vi "communicateWithAnalyzer.vi"(8 "ErrorIn":errorcluster, 11 "QueuesIn":T1) -> (0 "ErrorOut":errorcluster, 3 "QueuesOut":T1)   [LabVIEW 2019]
uses:
  utilities/Queues.ctl
  GUIVIs/GUIOutput.ctl
  MobileAnalyzer/mainVIs/analyzeAccelerationDataVIs/AccelerationDataFrames.ctl
  MobileAnalyzer/mainVIs/analyzeAccelerationDataVIs/AnalyzedVibrationsData.ctl
  MobileAnalyzer/mainVIs/analyzeAccelerationDataVIs/calculateFaultIndicatorsVIs/FaultDetections.ctl
  MobileAnalyzer/mainVIs/analyzeAccelerationDataVIs/calculateFaultIndicatorsVIs/ParameterFaultDetection.ctl
  MobileAnalyzer/mainVIs/analyzeAccelerationDataVIs/calculateFaultIndicatorsVIs/FaultParameter.ctl
  MobileAnalyzer/mainVIs/analyzeAccelerationDataVIs/calculateFaultIndicatorsVIs/FrequencyFaultDetection.ctl
  masterVIs/Command.ctl
  MobileAnalyzer/mainVIs/TDMSmanagerVIs/TDMSAnalyzerData.ctl
  MobileAnalyzer/mainVIs/TDMSmanagerVIs/TDMSAnalyzerDataType.ctl
  communicateWithAnalyzerVIs/CommunicateWithAnalyzerState.ctl
  MobileAnalyzer/mainVIs/AmasterVIs/ACommand.ctl
  masterVIs/Thread.ctl
  <vilib>/dex/Stream Element Allocation Mode.ctl
  communicateWithAnalyzerVIs/ReceiverData.ctl
  communicateWithAnalyzerVIs/ReceiverDataType.ctl
  MobileAnalyzer/mainVIs/UIVIs/UIOutput.ctl
  communicateWithAnalyzerVIs/SenderData.ctl
  communicateWithAnalyzerVIs/SenderDataType.ctl
  MobileAnalyzer/mainVIs/utilities/FGVAction.ctl
panel:
  in  "Connect":bool
  in  "SenderConnected":bool
  in  "ReceiverConnected":bool
  in  "Exit":bool
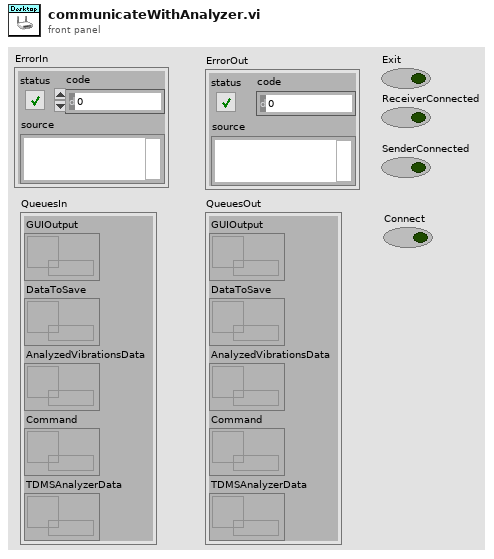
[diagram p1: front panel]
types:
  T1 = typedef "Queues.ctl" = cluster{"GUIOutput":refnum<queue>, "DataToSave":refnum<queue>, "AnalyzedVibrationsData":refnum<queue>, "Command":refnum<queue>, "TDMSAnalyzerData":refnum<queue>}
  T2 = typedef "ACommand.ctl" = enum16{"None", "Start", "Stop", "Restart", "SendFilesData", "DeleteAllData"}
  T3 = typedef "Command.ctl" = enum16{"None", "Connect", "Start", "Stop", "RestartAnalyzer", "Exit", "OpenDataFile", "CanBegin", "FileToSaveSettings", "AnalyzerSettings", "DownloadDataDialog", "DownloadData", "DeleteData"}
  T4 = typedef "Thread.ctl" = enum16{"GUI", "communicateWithAnalyzer", "saveDataToTDMS"}
  T5 = typedef "CommunicateWithAnalyzerState.ctl" = enum16{"Idle", "Connect", "Communicate", "Disconnect"}
  T6 = typedef "FGVAction.ctl" = enum16{"Read", "Write"}
  T7 = typedef "SenderDataType.ctl" = enum16{"Command", "AnalysisSettings"}
  T8 = typedef "SenderData.ctl" = cluster{"SenderDataType":T7, "Data":string}
  T9 = typedef "Stream Element Allocation Mode.ctl" = u32
  T10 = typedef "DesktopAppSettings.ctl" = cluster{"MobileAnalyzer IP":string, "Network Stream Timeout Code":i32, "Endpoint Destroyed Code":i32, "Save to file?":bool, "All threads":T4[], "Connected":bool, "AnalysisSettings":T11}
  T11 = typedef "AnalysisSettings.ctl" = cluster{"Fault Thresholds":T12, "Analysis series name":string, "Save data analysis?":bool}
  T12 = typedef "Thresholds.ctl" = cluster{"Parameters labels":T13[], "Parameters thresholds":dbl[], "Freqs and thresholds":dbl[][]}
  T13 = typedef "FaultParameter.ctl" = enum16{"Kurtosis", "RMS"}
  T14 = typedef "GUIOutput.ctl" = cluster{"Aquiring data":bool, "AnalyzerError":errorcluster, "FIFO overflow":bool, "Analyzing data":bool, "Connected":bool}
  T15 = typedef "ReceiverData.ctl" = cluster{"ReceiverDataType":T16, "Data":string}
  T16 = typedef "ReceiverDataType.ctl" = enum16{"UIOutput", "AnalyzedVibrationsData", "TDMSFiles"}
  T17 = typedef "UIOutput.ctl" = cluster{"Aquiring data":bool, "AnalyzerError":errorcluster, "FIFO overflow":bool, "Analyzing data":bool}
  T18 = typedef "AnalyzedVibrationsData.ctl" = cluster{"AccelerationDataFrames":T19, "Fault detections":T20}
  T19 = typedef "AccelerationDataFrames.ctl" = cluster{"AccelerationData":waveform(dbl)[], "Amplitudes":cluster{"f0":dbl, "df":dbl, "real part":dbl[]}[], "Phases":cluster{"f0":dbl, "df":dbl, "imaginary part":dbl[]}[]}
  T20 = typedef "FaultDetections.ctl" = cluster{"Parameters fault detection":T21[], "Frequencies fault detection":T22[]}
  T21 = typedef "ParameterFaultDetection.ctl" = cluster{"Axes Values":dbl[], "Axes Fault Detection":bool[], "Parameter Label":T13}
  T22 = typedef "FrequencyFaultDetection.ctl" = cluster{"Axes Values":dbl[], "Axes Fault Detection":bool[], "Frequency":dbl}
  T23 = typedef "TDMSAnalyzerData.ctl" = cluster{"TDMSAnalyzerDataType":T24, "group name out":string, "channel name(s) out":string[], "data":waveform(dbl)[], "File name":string}
  T24 = typedef "TDMSAnalyzerDataType.ctl" = enum16{"FileDataStart", "FileGroup", "FileDataStop", "NewFile", "EndOfFile"}
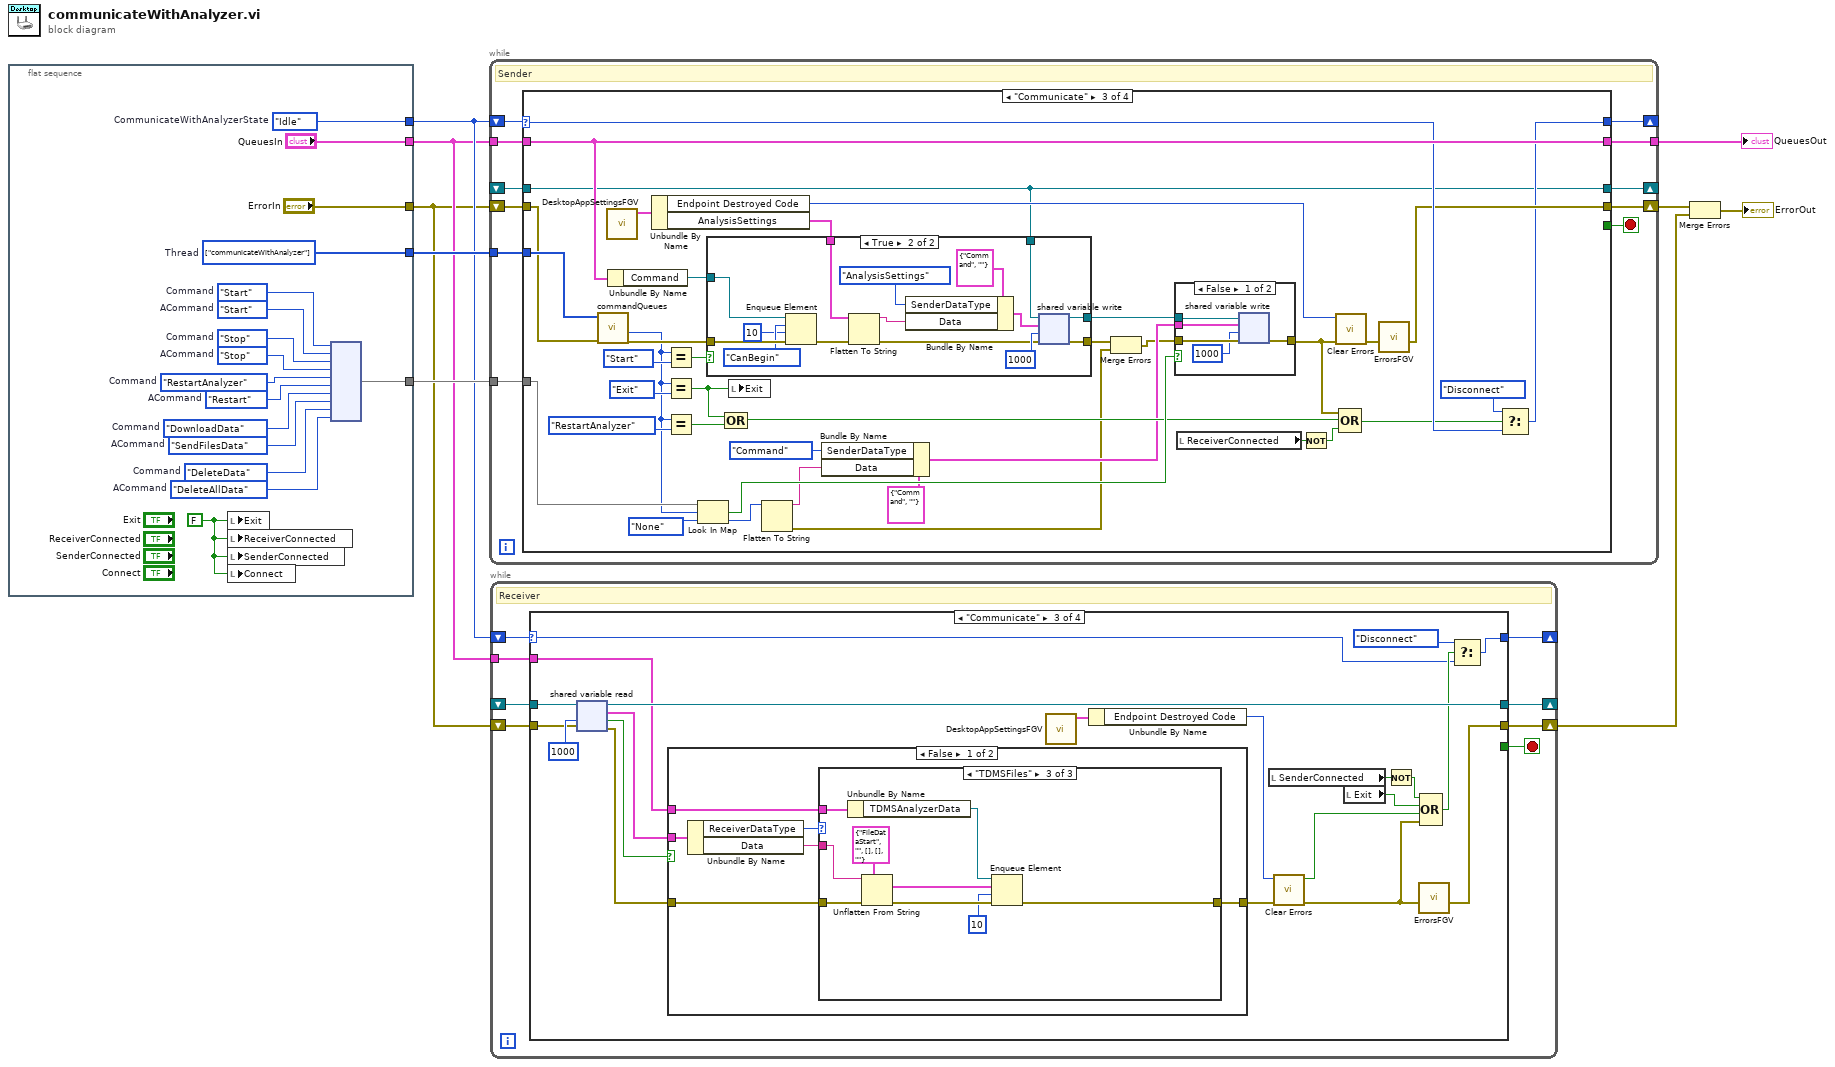
[diagram p0: block diagram]
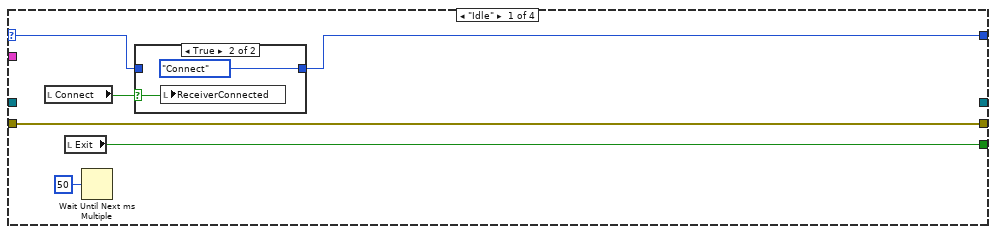
[diagram p2: hidden frame]
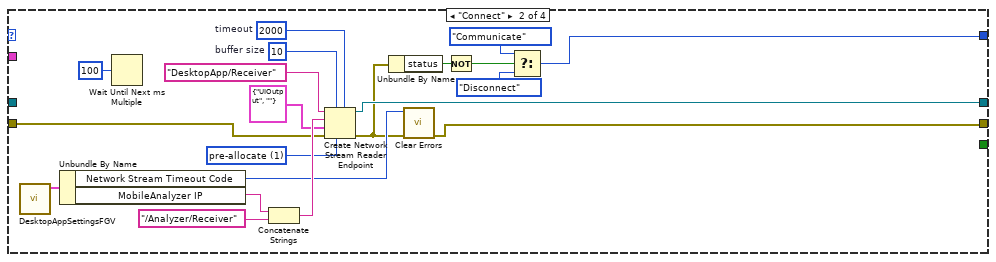
[diagram p4: hidden frame]
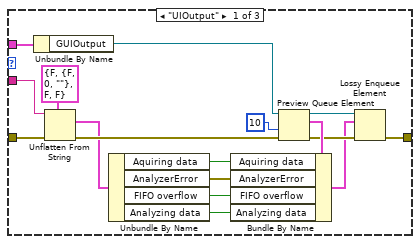
[diagram p5: hidden frame]
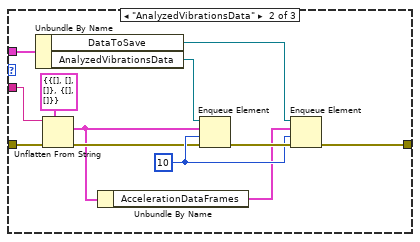
[diagram p6: hidden frame]
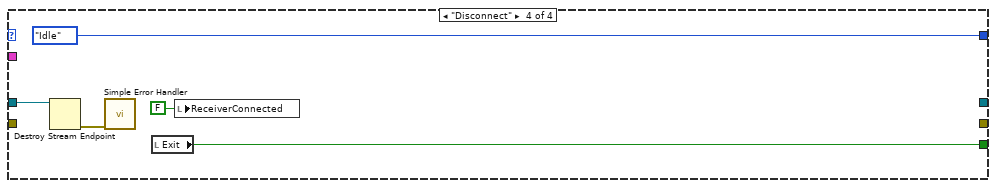
[diagram p8: hidden frame]
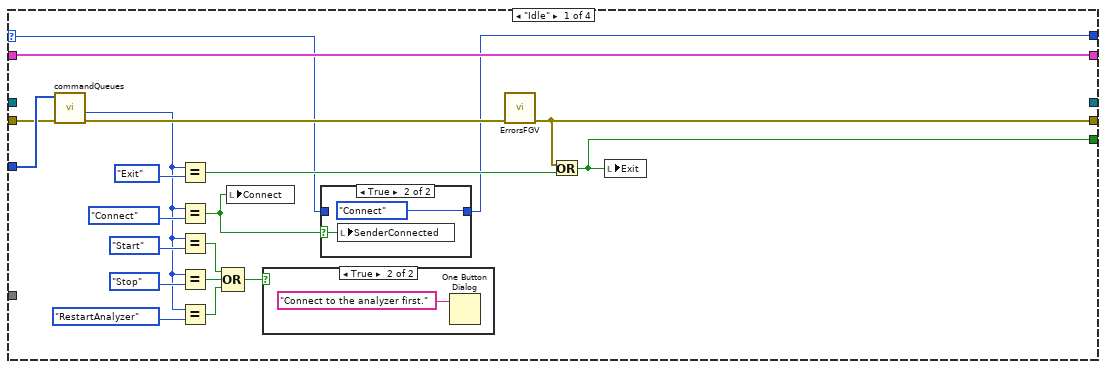
[diagram p9: hidden frame]
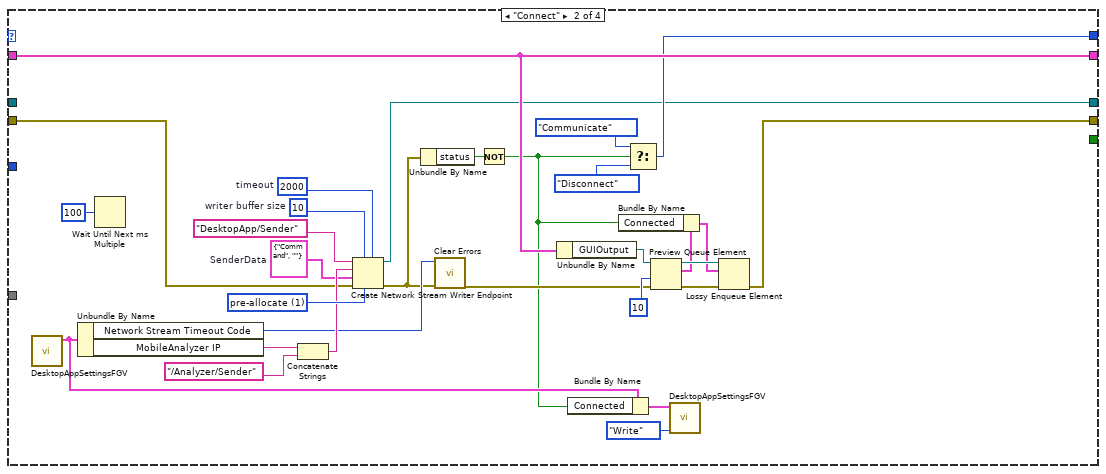
[diagram p12: hidden frame]
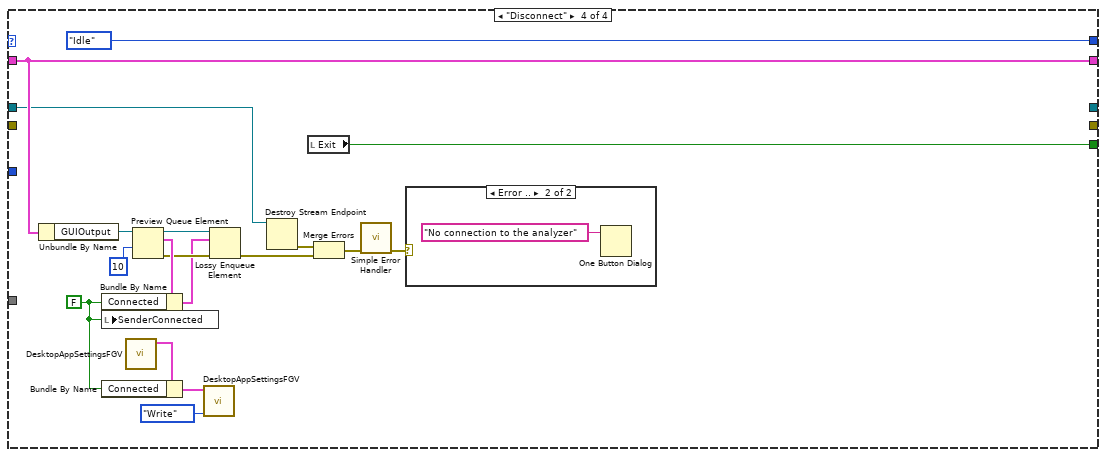
[diagram p15: hidden frame]
diagram:
  n1 = flat-sequence {
    tunnel: [w16] -> w6
    tunnel: ["QueuesIn"] -> w5
    tunnel: [w18] -> w8
    tunnel: [w17] -> w7
    tunnel: ["ErrorIn"] -> w2
    frame #0 {
      w10 = ACommand."DeleteAllData"  # ACommand
      w11 = Command."DeleteData"  # Command
      w12 = ACommand."SendFilesData"  # ACommand
      w13 = Command."DownloadData"  # Command
      w14 = FALSE ("Exit")
      w17 = T4[] [enum."communicateWithAnalyzer"] items=["GUI", "communicateWithAnalyzer", "saveDataToTDMS"]  # Thread
      w21 = Command."RestartAnalyzer"  # Command
      w22 = ACommand."Restart"  # ACommand
      w19 = Command."Stop"  # Command
      w20 = ACommand."Stop"  # ACommand
      w23 = Command."Start"  # Command
      w24 = ACommand."Start"  # ACommand
      w16 = CommunicateWithAnalyzerState."Idle"  # CommunicateWithAnalyzerState
      n2 = local write "Exit"(w14) -> ()
      n3 = local write "ReceiverConnected"(w14) -> ()
      n4 = local write "SenderConnected"(w14) -> ()
      n5 = local write "Connect"(w14) -> ()
      n6 = node(w23, w24, w19, w20, w21, w22, w13, w12, w11, w10) -> (w18:map{T3, T2})
    }
  }
  n7 = while {
    shift-right: [w28] -> w4
    shift-left: w2 -> [w30]
    shift-right: [w29] -> _
    shift-left: w6 -> [w31]
    tunnel: w5 -> [w35]
    tunnel: [w34] -> w9
    tunnel: w8 -> [w33]
    tunnel: w7 -> [w32]
    shift-right: [w26] -> _
    shift-left: _ -> [w27]
    stop <- w36 stop-if-true
    # "Sender"
    n8 = case shown="\"Communicate\"" w31 {
      selector: w31 -> [w38 _ w111 _]
      tunnel: [w40 _ _ w162] -> w36
      tunnel: w35 -> [w48 w83 w128 w163]
      tunnel: [w48 w83 w128 w163] -> w34
      tunnel: w33 -> [_ _ w114 _]
      tunnel: w32 -> [w47 _ w120 _]
      tunnel: w30 -> [w45 w74 w105 _]
      tunnel: [w37 w73 w106 CommunicateWithAnalyzerState."Idle" ("CommunicateWithAnalyzerState")] -> w29
      tunnel: [w42 w71 w107 _] -> w28
      tunnel: w27 -> [_ _ w100 w157]
      tunnel: [_ w72 w100 _] -> w26
      frame "Idle" {
        n9 = call "commandQueues.vi"("ErrorIn"=w45, "Threads"=w47) -> ("ErrorOut"=w44:errorcluster, "CommandOut"=w43:T3)  [unwired: 8 in]
        n10 = Equal?(x=w43, y=Command."Exit") -> (x = y?=w41:bool)
        n11 = Equal?(x=w43, y=Command."Connect") -> (x = y?=w39:bool)
        n12 = Equal?(x=w43, y=Command."Start") -> (x = y?=w50:bool)
        n13 = Equal?(x=w43, y=Command."Stop") -> (x = y?=w51:bool)
        n14 = Equal?(x=w43, y=Command."RestartAnalyzer") -> (x = y?=w49:bool)
        n15 = Compound Arithmetic op=OR(w50, w51, w49) -> (w46:bool)
        n16 = local write "Connect"(w39) -> ()
        n17 = case shown="True" w46 {
          frame False {
          }
          frame True {
            n18 = One Button Dialog(message="Connect to the analyzer first." ("source")) -> ()  [unwired: 1 in, 1 out]
          }
        }
        n19 = case shown="True" w39 {
          selector: w39 -> [_ w59]
          tunnel: [w57 CommunicateWithAnalyzerState."Connect" ("CommunicateWithAnalyzerState")] -> w37
          tunnel: w38 -> [w57 _]
          frame False {
          }
          frame True {
            n20 = local write "SenderConnected"(w59) -> ()
          }
        }
        n21 = call "ErrorsFGV.vi"("CriticalErrorIn"=w44) -> ("CriticalErrorOut"=w42:errorcluster)  [unwired: 7 in, 3 out]
        n22 = Or(x=w42, y=w41) -> (x .or. y?=w40:bool)
        n23 = local write "Exit"(w40) -> ()
      }
      frame "Connect" {
        w65 = T8 {"SenderDataType"=enum."Command", "Data"=""}  # SenderData
        w79 = 2000  # timeout
        w80 = 10  # writer buffer size
        w82 = T9 1 items=["allocate as needed", "pre-allocate"] ("element allocation mode")
        n24 = call "DesktopAppSettingsFGV.vi"() -> ("DesktopAppSettingsOut"=w64:T10)  [unwired: 11 in]
        n25 = Unbundle By Name(w64) -> ("Network Stream Timeout Code"=w75:i32, "MobileAnalyzer IP"=w76:string)
        n26 = Wait Until Next ms Multiple(millisecond multiple=u32 100) -> ()  [unwired: 1 out]
        n27 = Concatenate Strings(w76, "/Analyzer/Sender") -> (w77:string)
        n28 = Create Network Stream Writer Endpoint(5:w79, 6:w82, 7:w80, 8:w74, 9:w65, 10:w77, 11:"DesktopApp/Sender" ("writer name")) -> (0:w67:errorcluster, 3:w72:refnum<k21>)
        n29 = Unbundle By Name(w67) -> ("status"=w68:bool)
        n30 = call <vilib>:"Clear Errors.vi"("error in (no error)"=w67, "specific error code to clear (0: all)"=w75) -> ("error out"=w85:errorcluster)  [unwired: 4 in, 1 out]
        n31 = Not(x=w68) -> (.not. x?=w63:bool)
        n32 = Unbundle By Name(w83) -> ("GUIOutput"=w84:refnum<queue>)
        n33 = Bundle By Name(cluster=w64, "Connected"=w63) -> (w62:T10)
        n34 = Select(t=CommunicateWithAnalyzerState."Communicate" ("CommunicateWithAnalyzerState"), s=w63, f=CommunicateWithAnalyzerState."Disconnect" ("CommunicateWithAnalyzerState")) -> (s? t:f=w73:T5)
        n35 = Preview Queue Element(queue=w84, timeout in ms (-1)=10, error in (no error)=w85) -> (queue out=w87:refnum<queue>, element=w70:T14, error out=w86:errorcluster)  [unwired: 1 out]
        n36 = Bundle By Name(cluster=w70, "Connected"=w63) -> (w69:T14)
        n37 = call "DesktopAppSettingsFGV.vi"("FGVAction (Read)"=FGVAction."Write", "DesktopAppSettingsIn"=w62) -> ()  [unwired: 9 in, 1 out]
        n38 = Lossy Enqueue Element(queue=w87, element=w69, error in (no error)=w86) -> (error out=w71:errorcluster)  [unwired: 3 out]
      }
      frame "Communicate" {
        n39 = call "commandQueues.vi"("ErrorIn"=w105, "Threads"=w120) -> ("ErrorOut"=w117:errorcluster, "CommandOut"=w103:T3)  [unwired: 8 in]
        n40 = call "DesktopAppSettingsFGV.vi"() -> ("DesktopAppSettingsOut"=w125:T10)  [unwired: 11 in]
        n41 = Unbundle By Name(w128) -> ("Command"=w116:refnum<queue>)
        n42 = Unbundle By Name(w125) -> ("Endpoint Destroyed Code"=w113:i32, "AnalysisSettings"=w98:T11)
        n43 = Equal?(x=w103, y=Command."Start") -> (x = y?=w115:bool)
        n44 = Equal?(x=w103, y=Command."Exit") -> (x = y?=w122:bool)
        n45 = Equal?(x=w103, y=Command."RestartAnalyzer") -> (x = y?=w123:bool)
        n46 = Look In Map(map=w114, key=w103, default value=ACommand."None") -> (key not found?=w127:bool, value=w94:T2)
        n47 = case shown="True" w115 {
          tunnel: [w130 w141] -> w118
          tunnel: w117 -> [w130 w145]
          tunnel: w116 -> [_ w144]
          tunnel: w100 -> [w129 w140]
          tunnel: [w129 w139] -> w99
          tunnel: w98 -> [_ w132]
          frame False {
          }
          frame True {
            n48 = Enqueue Element(queue=w144, element=Command."CanBegin", timeout in ms (-1)=10, error in (no error)=w145) -> (error out=w134:errorcluster)  [unwired: 2 out]
            n49 = Flatten To String(anything=w132, error in (no error)=w134) -> (data string=w131:string, error out=w133:errorcluster)  [unwired: 2 in, 1 out]
            n50 = Bundle By Name(cluster=T8 {"SenderDataType"=enum."Command", "Data"=""} ("SenderData"), "SenderDataType"=SenderDataType."AnalysisSettings", "Data"=w131) -> (w135:T8)
            n51 = shared-variable-write(w140, w133, w135, 1000 ("timeout ms (-1)")) -> (w139:refnum<k21>, w141:errorcluster)  [unwired: 1 out]
          }
        }
        n52 = Compound Arithmetic op=OR(w122, w123) -> (w121:bool)
        n53 = local write "Exit"(w122) -> ()
        n54 = Flatten To String(anything=w94) -> (data string=w93:string, error out=w92:errorcluster)  [unwired: 3 in, 1 out]
        n55 = Bundle By Name(cluster=T8 {"SenderDataType"=enum."Command", "Data"=""} ("SenderData"), "SenderDataType"=SenderDataType."Command", "Data"=w93) -> (w95:T8)
        n56 = Merge Errors(w118, w92) -> (w91:errorcluster)
        n57 = case shown="False" w127 {
          tunnel: w95 -> [w150 _]
          tunnel: w91 -> [w149 w151]
          tunnel: [w148 w151] -> w112
          tunnel: w99 -> [w146 _]
          frame False {
            n58 = shared-variable-write(w146, w149, w150, 1000 ("timeout ms (-1)")) -> (w148:errorcluster)  [unwired: 2 out]
          }
          frame True {
          }
        }
        n59 = local read "ReceiverConnected"() -> (w102:bool)
        n60 = Not(x=w102) -> (.not. x?=w101:bool)
        n61 = call <vilib>:"Clear Errors.vi"("error in (no error)"=w112, "specific error code to clear (0: all)"=w113) -> ("error out"=w108:errorcluster)  [unwired: 4 in, 1 out]
        n62 = Compound Arithmetic op=OR(w112, w121, w101) -> (w109:bool)
        n63 = call "ErrorsFGV.vi"("InternalErrorIn"=w108) -> ("InternalErrorOut"=w107:errorcluster)  [unwired: 7 in, 3 out]
        n64 = Select(t=CommunicateWithAnalyzerState."Disconnect", s=w109, f=w111) -> (s? t:f=w106:T5)
      }
      frame "Disconnect" {
        w154 = FALSE ("Device working")
        n65 = Unbundle By Name(w163) -> ("GUIOutput"=w164:refnum<queue>)
        n66 = local write "SenderConnected"(w154) -> ()
        n67 = call "DesktopAppSettingsFGV.vi"() -> ("DesktopAppSettingsOut"=w152:T10)  [unwired: 11 in]
        n68 = Bundle By Name(cluster=w152, "Connected"=w154) -> (w153:T10)
        n69 = Preview Queue Element(queue=w164, timeout in ms (-1)=10) -> (queue out=w168:refnum<queue>, element=w169:T14, error out=w167:errorcluster)  [unwired: 1 in, 1 out]
        n70 = Bundle By Name(cluster=w169, "Connected"=w154) -> (w166:T14)
        n71 = call "DesktopAppSettingsFGV.vi"("FGVAction (Read)"=FGVAction."Write", "DesktopAppSettingsIn"=w153) -> ()  [unwired: 9 in, 1 out]
        n72 = Lossy Enqueue Element(queue=w168, element=w166, error in (no error)=w167) -> (error out=w158:errorcluster)  [unwired: 3 out]
        n73 = Destroy Stream Endpoint(11:w157) -> (0:w161:errorcluster)  [unwired: 1 in]
        n74 = local read "Exit"() -> (w162:bool)
        n75 = Merge Errors(w161, w158) -> (w160:errorcluster)
        n76 = call <vilib>:"Simple Error Handler.vi"("error in (no error)"=w160) -> ("error out"=w156:errorcluster)  [unwired: 4 in, 4 out]
        n77 = case shown="Error .." w156 {
          frame No Error {
          }
          frame Error {
            n78 = One Button Dialog(message="No connection to the analyzer") -> ()  [unwired: 1 in, 1 out]
          }
        }
      }
    }
  }
  "QueuesOut" <- w9
  n79 = while {
    shift-right: [w174] -> _
    shift-left: w6 -> [w176]
    shift-right: [w177] -> w3
    shift-left: w2 -> [w178]
    tunnel: w5 -> [w175]
    shift-right: [w172] -> _
    shift-left: _ -> [w171]
    stop <- w173 stop-if-true
    # "Receiver"
    n80 = case shown="\"Communicate\"" w176 {
      selector: w176 -> [w180 _ w211 _]
      tunnel: w178 -> [w182 w198 w225 _]
      tunnel: [w182 w192 w214 _] -> w177
      tunnel: w175 -> [_ _ w221 _]
      tunnel: [w179 w193 w212 CommunicateWithAnalyzerState."Idle" ("CommunicateWithAnalyzerState")] -> w174
      tunnel: [w184 _ _ w274] -> w173
      tunnel: [_ w197 w226 _] -> w172
      tunnel: w171 -> [_ _ w227 w276]
      frame "Idle" {
        n81 = local read "Connect"() -> (w181:bool)
        n82 = local read "Exit"() -> (w184:bool)
        n83 = Wait Until Next ms Multiple(millisecond multiple=u32 50) -> ()  [unwired: 1 out]
        n84 = case shown="True" w181 {
          selector: w181 -> [_ w186]
          tunnel: [w185 CommunicateWithAnalyzerState."Connect" ("t")] -> w179
          tunnel: w180 -> [w185 _]
          frame False {
          }
          frame True {
            n85 = local write "ReceiverConnected"(w186) -> ()
          }
        }
      }
      frame "Connect" {
        w204 = 2000  # timeout
        w202 = 10  # buffer size
        w203 = T9 1 items=["allocate as needed", "pre-allocate"] ("element allocation mode")
        n86 = call "DesktopAppSettingsFGV.vi"() -> ("DesktopAppSettingsOut"=w206:T10)  [unwired: 11 in]
        n87 = Unbundle By Name(w206) -> ("Network Stream Timeout Code"=w196:i32, "MobileAnalyzer IP"=w207:string)
        n88 = Wait Until Next ms Multiple(millisecond multiple=u32 100) -> ()  [unwired: 1 out]
        n89 = Concatenate Strings(w207, "/Analyzer/Receiver") -> (w205:string)
        n90 = Create Network Stream Reader Endpoint(5:w204, 6:w203, 7:w202, 8:w198, 9:T15 {"ReceiverDataType"=enum."UIOutput", "Data"=""} ("ReceiverData"), 10:w205, 11:"DesktopApp/Receiver" ("writer name")) -> (0:w190:errorcluster, 3:w197:refnum<k21>)
        n91 = Unbundle By Name(w190) -> ("status"=w191:bool)
        n92 = call <vilib>:"Clear Errors.vi"("error in (no error)"=w190, "specific error code to clear (0: all)"=w196) -> ("error out"=w192:errorcluster)  [unwired: 4 in, 1 out]
        n93 = Not(x=w191) -> (.not. x?=w189:bool)
        n94 = Select(t=CommunicateWithAnalyzerState."Communicate" ("CommunicateWithAnalyzerState"), s=w189, f=CommunicateWithAnalyzerState."Disconnect" ("CommunicateWithAnalyzerState")) -> (s? t:f=w193:T5)
      }
      frame "Communicate" {
        n95 = shared-variable-read(w227, w225, 1000 ("timeout ms (-1)")) -> (w226:refnum<k21>, w222:errorcluster, w223:bool, w224:T15)
        n96 = case shown="False" w223 {
          tunnel: w224 -> [w234 _]
          tunnel: w222 -> [w231 w273]
          tunnel: w221 -> [w230 _]
          tunnel: [w229 w273] -> w219
          frame False {
            n97 = Unbundle By Name(w234) -> ("ReceiverDataType"=w233:T16, "Data"=w232:string)
            n98 = case shown="\"TDMSFiles\"" w233 {
              tunnel: w232 -> [w237 w254 w270]
              tunnel: w231 -> [w239 w256 w271]
              tunnel: w230 -> [w251 w263 w269]
              tunnel: [w240 w260 w267] -> w229
              frame "UIOutput" {
                n99 = Unbundle By Name(w251) -> ("GUIOutput"=w242:refnum<queue>)
                n100 = Unflatten From String(type=T17 {"Aquiring data"=FALSE, "AnalyzerError"={"status"=FALSE, "code"=0, "source"=""}, "FIFO overflow"=FALSE, "Analyzing data"=FALSE} ("UIOutput"), binary string=w237, error in (no error)=w239) -> (value=w235:T17, error out=w238:errorcluster)  [unwired: 2 in, 1 out]
                n101 = Unbundle By Name(w235) -> ("Aquiring data"=w243:bool, "AnalyzerError"=w250:errorcluster, "FIFO overflow"=w245:bool, "Analyzing data"=w244:bool)
                n102 = Preview Queue Element(queue=w242, timeout in ms (-1)=10, error in (no error)=w238) -> (queue out=w249:refnum<queue>, element=w248:T14, error out=w247:errorcluster)  [unwired: 1 out]
                n103 = Bundle By Name(cluster=w248, "Aquiring data"=w243, "AnalyzerError"=w250, "FIFO overflow"=w245, "Analyzing data"=w244) -> (w246:T14)
                n104 = Lossy Enqueue Element(queue=w249, element=w246, error in (no error)=w247) -> (error out=w240:errorcluster)  [unwired: 3 out]
              }
              frame "AnalyzedVibrationsData" {
                w258 = 10 ("timeout in ms (-1)")
                n105 = Unbundle By Name(w263) -> ("DataToSave"=w259:refnum<queue>, "AnalyzedVibrationsData"=w262:refnum<queue>)
                n106 = Unflatten From String(type=T18 {"AccelerationDataFrames"={"AccelerationData"=[], "Amplitudes"=[], "Phases"=[]}, "Fault detections"={"Parameters fault detection"=[], "Frequencies fault detection"=[]}} ("AnalyzedVibrationsData"), binary string=w254, error in (no error)=w256) -> (value=w252:T18, error out=w255:errorcluster)  [unwired: 2 in, 1 out]
                n107 = Unbundle By Name(w252) -> ("AccelerationDataFrames"=w257:T19)
                n108 = Enqueue Element(queue=w262, element=w252, timeout in ms (-1)=w258, error in (no error)=w255) -> (error out=w261:errorcluster)  [unwired: 2 out]
                n109 = Enqueue Element(queue=w259, element=w257, timeout in ms (-1)=w258, error in (no error)=w261) -> (error out=w260:errorcluster)  [unwired: 2 out]
              }
              frame "TDMSFiles" {
                n110 = Unbundle By Name(w269) -> ("TDMSAnalyzerData"=w266:refnum<queue>)
                n111 = Unflatten From String(type=T23 {"TDMSAnalyzerDataType"=enum."FileDataStart", "group name out"="", "channel name(s) out"=[], "data"=[], "File name"=""} ("TDMSAnalyzerData"), binary string=w270, error in (no error)=w271) -> (value=w265:T23, error out=w268:errorcluster)  [unwired: 2 in, 1 out]
                n112 = Enqueue Element(queue=w266, element=w265, timeout in ms (-1)=10, error in (no error)=w268) -> (error out=w267:errorcluster)  [unwired: 2 out]
              }
            }
          }
          frame True {
          }
        }
        n113 = call "DesktopAppSettingsFGV.vi"() -> ("DesktopAppSettingsOut"=w220:T10)  [unwired: 11 in]
        n114 = Unbundle By Name(w220) -> ("Endpoint Destroyed Code"=w218:i32)
        n115 = local read "SenderConnected"() -> (w209:bool)
        n116 = call <vilib>:"Clear Errors.vi"("error in (no error)"=w219, "specific error code to clear (0: all)"=w218) -> ("error out"=w217:errorcluster, "specific error cleared?"=w215:bool)  [unwired: 4 in]
        n117 = local read "Exit"() -> (w216:bool)
        n118 = Not(x=w209) -> (.not. x?=w208:bool)
        n119 = call "ErrorsFGV.vi"("InternalErrorIn"=w217) -> ("InternalErrorOut"=w214:errorcluster)  [unwired: 7 in, 3 out]
        n120 = Compound Arithmetic op=OR(w208, w216, w215, w217) -> (w213:bool)
        n121 = Select(t=CommunicateWithAnalyzerState."Disconnect", s=w213, f=w211) -> (s? t:f=w212:T5)
      }
      frame "Disconnect" {
        n122 = Destroy Stream Endpoint(11:w276) -> (0:w275:errorcluster)  [unwired: 1 in]
        n123 = call <vilib>:"Simple Error Handler.vi"("error in (no error)"=w275) -> ()  [unwired: 4 in, 5 out]
        n124 = local read "Exit"() -> (w274:bool)
        n125 = local write "ReceiverConnected"(FALSE ("ReceiverConnected")) -> ()
      }
    }
  }
  n126 = Merge Errors(w4, w3) -> (→"ErrorOut":errorcluster)
